vi "Get Sim LMS Vector 5.vi"(8 "Compass":dbl, 9 "GPS Data":dbl[](array[numeric])=[37.1526, 81.2675, 7.3], 11 "Obst Lats and Longs":cluster{"Obst Lats":dbl[], "Obst Longs":dbl[]}={"Obst Lats"=[0.0, 0.0, 0.0, 37.152613, 37.152608, 37.152615, 37.152603, 37.152779, 37.152868, 37.152484], "Obst Longs"=[0.0, 0.0, 0.0, 81.267502, 81.267507, 81.2675, 81.267512, 81.267301, 81.267913, 81.26772]} {"Obst Longs" format="%#_8g"; "Obst Lats" format="%#_8g"}) -> (2 "LMS Vector":dbl[](array[numeric]))   [LabVIEW 2014]
panel:
  out "num of obs":dbl
  out "Angle of obstacle":dbl[](array[numeric])
  out "Dist to obstacle":dbl[](array[numeric])
  # "Get Simulated LMS and make it into LMS Vector"
  # "Get Sim LMS Vector 5.vi"
  # "Inputs:"
  # "Outputs:"
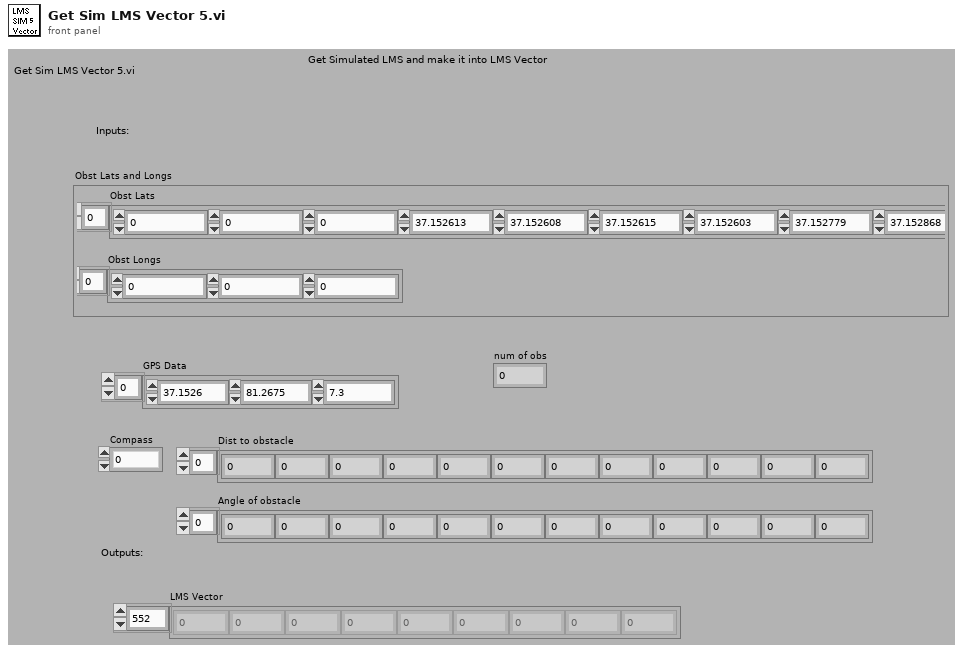
[diagram p1: front panel]
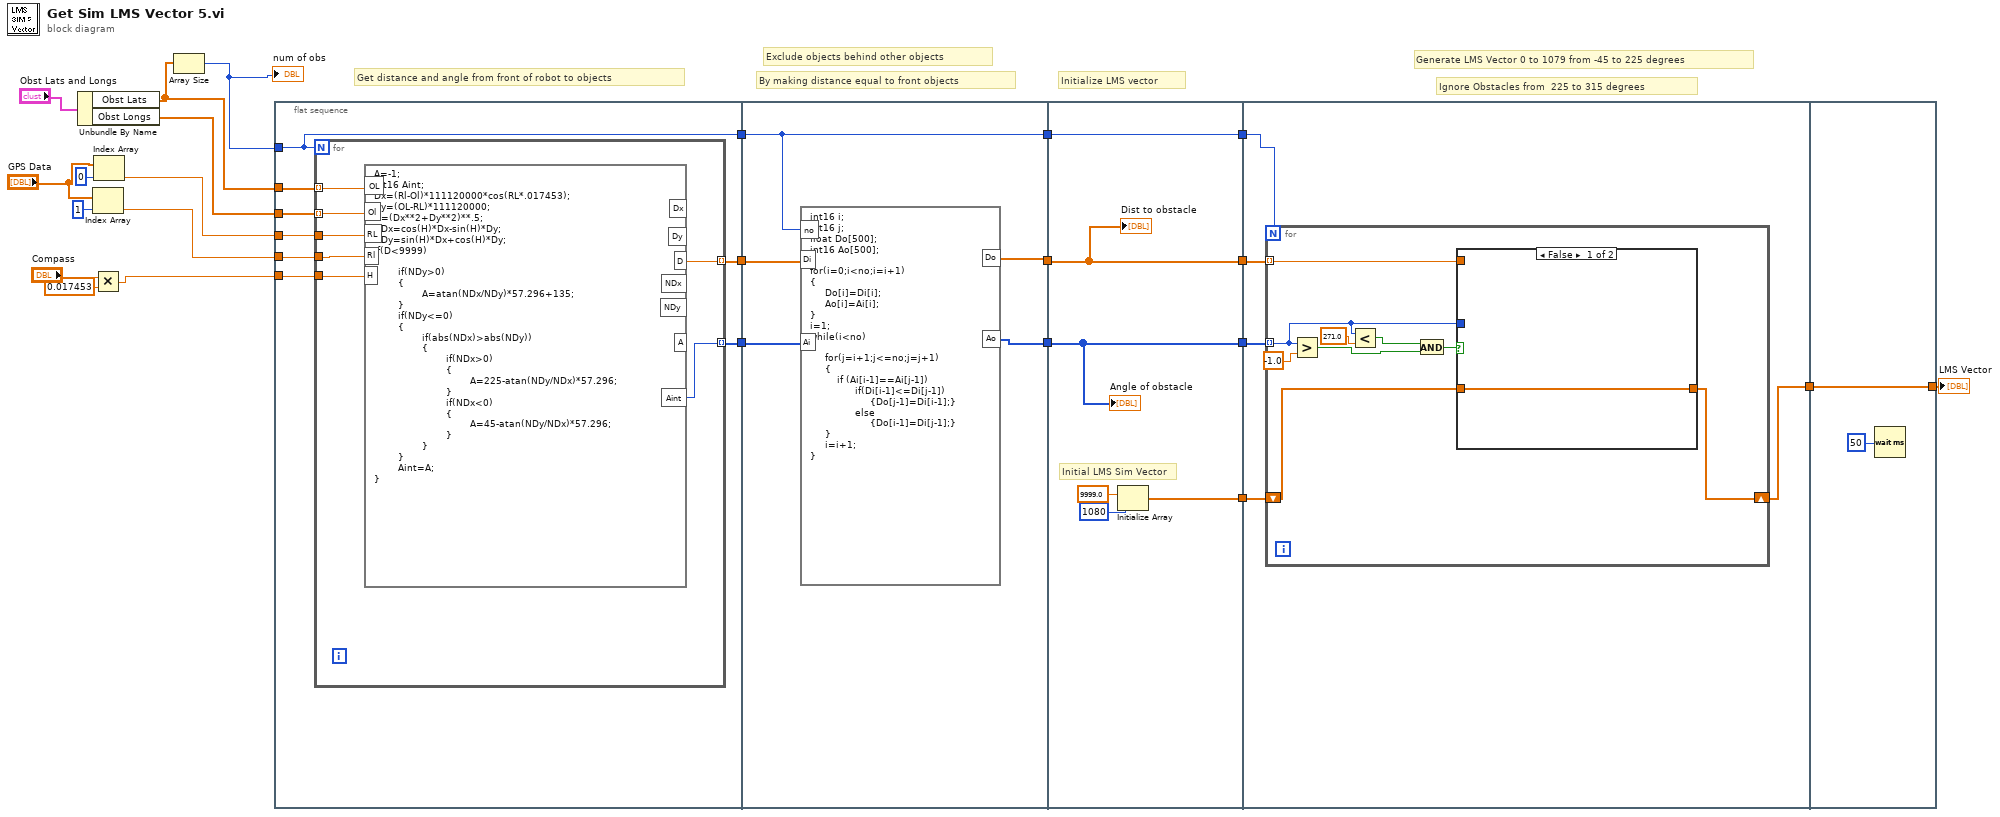
[diagram p0: block diagram]
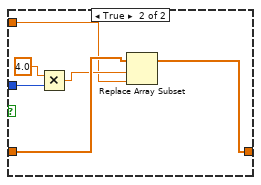
[diagram p2: hidden frame]
diagram:
  # "Ignore Obstacles from  225 to 315 degrees"
  # "Generate LMS Vector 0 to 1079 from -45 to 225 degrees"
  # "By making distance equal to front objects"
  # "Initialize LMS vector"
  # "Exclude objects behind other objects"
  # "Get distance and angle from front of robot to objects"
  n1 = Unbundle By Name("Obst Lats and Longs") -> ("Obst Lats"=w23:dbl[], "Obst Longs"=w22:dbl[])
  n2 = Index Array(array="GPS Data", index=1) -> (element=w17:dbl)
  n3 = Multiply(x="Compass", y=0.017453) -> (x*y=w14:dbl)
  n4 = Index Array(array="GPS Data", index=0) -> (element=w18:dbl)
  n5 = Array Size(array=w23) -> (size(s)=w8:i32)
  "num of obs" <- w8
  n6 = flat-sequence {
    tunnel: w8 -> [w27]
    tunnel: w23 -> [w32]
    tunnel: w22 -> [w31]
    tunnel: w18 -> [w30]
    tunnel: w17 -> [w29]
    tunnel: w14 -> [w28]
    tunnel: [w27] -> w6
    tunnel: [w26] -> w4
    tunnel: [w25] -> w2
    tunnel: w6 -> [w40]
    tunnel: [w40] -> w5
    tunnel: w4 -> [w44]
    tunnel: [w42] -> w3
    tunnel: w2 -> [w43]
    tunnel: [w41] -> w1
    tunnel: [w48] -> w13
    tunnel: w5 -> [w48]
    tunnel: [w47] -> w12
    tunnel: w3 -> [w46]
    tunnel: [w46] -> w11
    tunnel: w1 -> [w45]
    tunnel: [w45] -> w10
    tunnel: w13 -> [w55]
    tunnel: w12 -> [w54]
    tunnel: w11 -> [w53]
    tunnel: w10 -> [w52]
    tunnel: [w51] -> w7
    tunnel: [w73] -> w9
    tunnel: w7 -> [w73]
    frame #0 {
      n7 = for {
        N: w27 -> [_]
        tunnel: w32 -> [w35] mode=indexing
        tunnel: w31 -> [w36] mode=indexing
        tunnel: w30 -> [w37]
        tunnel: w29 -> [w38]
        tunnel: w28 -> [w39]
        tunnel: [w33] -> w25 mode=indexing
        tunnel: [w34] -> w26 mode=indexing
        n8 = formula code="A=-1;\nint16 Aint;\nDx=(Rl-Ol)*111120000*cos(RL*.017453);\nDy=(OL-RL)*111120000;\nD=(Dx**2+Dy**2)**.5;\nNDx=cos(H)*Dx-sin(H)*Dy;\nNDy=sin(H)*Dx+cos(H)*Dy;\nif(D<9999)\n{\n        if(NDy>0)\n        {\n                A=atan(NDx/NDy)*57.296+135;\n        }\n        if(NDy<=0)\n        {\n                if(abs(NDx)>abs(NDy))\n                {\n                        if(NDx>0)\n                        {\n                                A=225-atan(NDy/NDx)*57.296;\n                        }\n                        if(NDx<0)\n                        {\n                                A=45-atan(NDy/NDx)*57.296;\n                        }\n                }\n        }\n        Aint=A;\n}"("OL"=w35, "Ol"=w36, "RL"=w37, "Rl"=w38, "H"=w39) -> ("D"=w34:dbl, "Aint"=w33:i16)  [unwired: 5 out]
      }
    }
    frame #1 {
      n9 = formula code="int16 i;\nint16 j;\nfloat Do[500];\nint16 Ao[500];\n\nfor(i=0;i<no;i=i+1)\n{\n     Do[i]=Di[i];\n     Ao[i]=Ai[i];\n}\ni=1;\nwhile(i<no)\n{\n     for(j=i+1;j<=no;j=j+1)\n     {\n         if (Ai[i-1]==Ai[j-1])\n               if(Di[i-1]<=Di[j-1])\n                    {Do[j-1]=Di[i-1];}\n               else\n                    {Do[i-1]=Di[j-1];}\n     }\n     i=i+1;\n}"("Di"=w44, "Ai"=w43, "no"=w40) -> ("Do"=w42:dbl[], "Ao"=w41:i16[])
    }
    frame #2 {
      # "Initial LMS Sim Vector"
      n10 = Initialize Array(9999.0 ("element"), 1080 ("dimension size")) -> (w47:dbl[])
      "Dist to obstacle" <- w46
      "Angle of obstacle" <- w45
    }
    frame #3 {
      n11 = for {
        N: w55 -> [_]
        tunnel: w53 -> [w63] mode=indexing
        tunnel: w52 -> [w61] mode=indexing
        shift-right: [w56] -> w51
        shift-left: w54 -> [w62]
        n12 = Greater?(x=w61, y=-1.0) -> (0:w58:bool)
        n13 = Less?(x=w61, y=271.0) -> (x < y?=w59:bool)
        n14 = And(x=w59, y=w58) -> (x .and. y?=w57:bool)
        n15 = case shown="False" w57 {
          tunnel: w63 -> [_ w67]
          tunnel: w61 -> [_ w71]
          tunnel: w62 -> [w65 w69]
          tunnel: [w65 w66] -> w56
          frame False {
          }
          frame True {
            n16 = Multiply(x=4.0, y=w71) -> (x*y=w68:dbl)
            n17 = Replace Array Subset(array=w69, new element=w67, index=w68) -> (w66:dbl[])
          }
        }
      }
    }
    frame #4 {
      n18 = Wait (ms)(milliseconds to wait=u32 50) -> ()  [unwired: 1 out]
    }
  }
  "LMS Vector" <- w9
